vi "New UTF-8 String.vi"(6 "error in":errorcluster, 9 "LabVIEW String":T1) -> (1 "UTF-8 String":refnum<class "UTF-8 String.lvclass">, 4 "error out":errorcluster)   [LabVIEW 2020, in "G-Unicode.lvlib" / "UTF-8 String.lvclass"]
doc: "Initializes a new UTF-8 string. <b>LabVIEW String</b> will be encoded as UTF-8 using the local codepage.\n\nIf you have a LabVIEW string which is already UTF-8 encoded, use <b>Write Raw UTF-8 String.vi</b> instead."
uses:
  UTF-8 String.lvclass
  Encoded UTF-8 String.ctl
  UTF-8 String.lvclass/UTF-8 String.ctl
  G-Unicode.lvlib
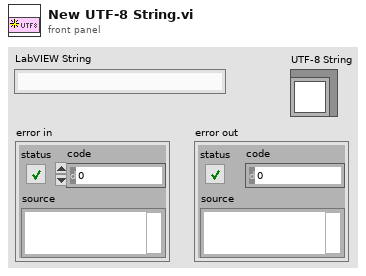
[diagram p1: front panel]
types:
  T1 = typedef "G-Unicode.lvlib/Encoded UTF-8 String.ctl" = string
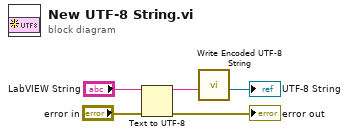
[diagram p0: block diagram]
diagram:
  n1 = Text to UTF-8(8:"error in", 11:"LabVIEW String") -> (0:→"error out":errorcluster, 3:w4:string)  [unwired: 1 in]
  n2 = call "Write Encoded UTF-8 String.vi"("Raw UTF-8 String"=w4) -> ("UTF-8 String"=→"UTF-8 String":refnum<class "UTF-8 String.lvclass">)  [unwired: 10 in]
